vi "NewSerialSource.vi"() -> (0 "Select Source 2":refnum<visa-resource-name>)   [LabVIEW 2010]
panel:
  in  "请选择使用的串口":refnum<visa-resource-name>
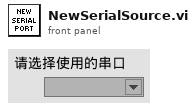
[diagram p1: front panel]
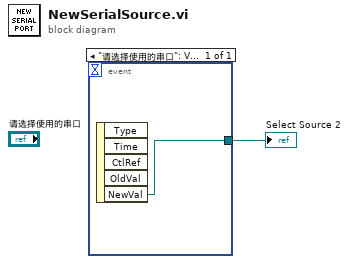
[diagram p0: block diagram]
diagram:
  n1 = event shown="[0] \"请选择使用的串口\": Value Change" {
    selector: _ -> [_]
    dyn-events: _ -> [_]
    timeout: _ -> [_]
    tunnel: [w2] -> w1
    event "请选择使用的串口": Value Change {
      n2 = event-data() -> ("NewVal"=w2:refnum<visa-resource-name>)  [unwired: 1 in, 4 out]
    }
  }
  "Select Source 2" <- w1
